vi "Final Shutdown.vi"(8 "error in (no error)":errorcluster, 11 "Main Controller in":refnum<class "Main Controller Actor.lvclass">) -> (0 "error out":errorcluster)   [LabVIEW 2021, in "Main Controller Actor.lvclass"]
uses:
  Main Controller Actor.lvclass
  Main Controller Actor.lvclass/Main Controller Actor.ctl
  Error Handler/API/Error Handler Actor API.lvclass
  Sprite Font/Sprite Font.lvclass
  Re-use Libraries/Minimal Actor Framework/Actors/Base Actor/API/Actor API.lvclass
  Task Scheduler/API/Task Scheduler Actor API.lvclass
  Element/Element.lvclass
  Globals.vi
  Re-use Libraries/Minimal Actor Framework/Actors/Base Actor/Actor/Actor.lvclass
  LabBASSMOD2/LabBASSMOD2.lvlib
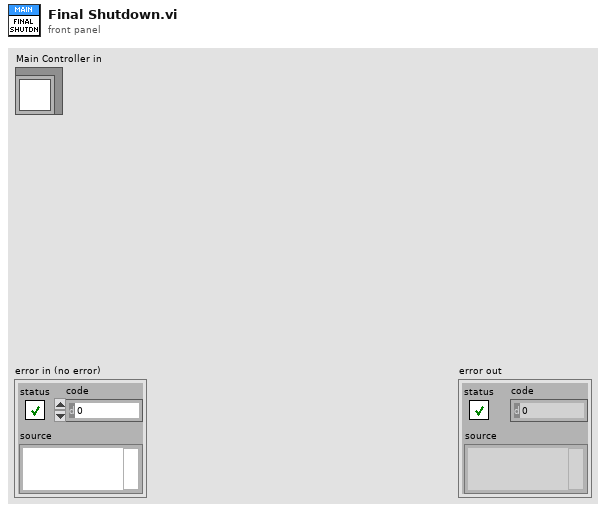
[diagram p1: front panel]
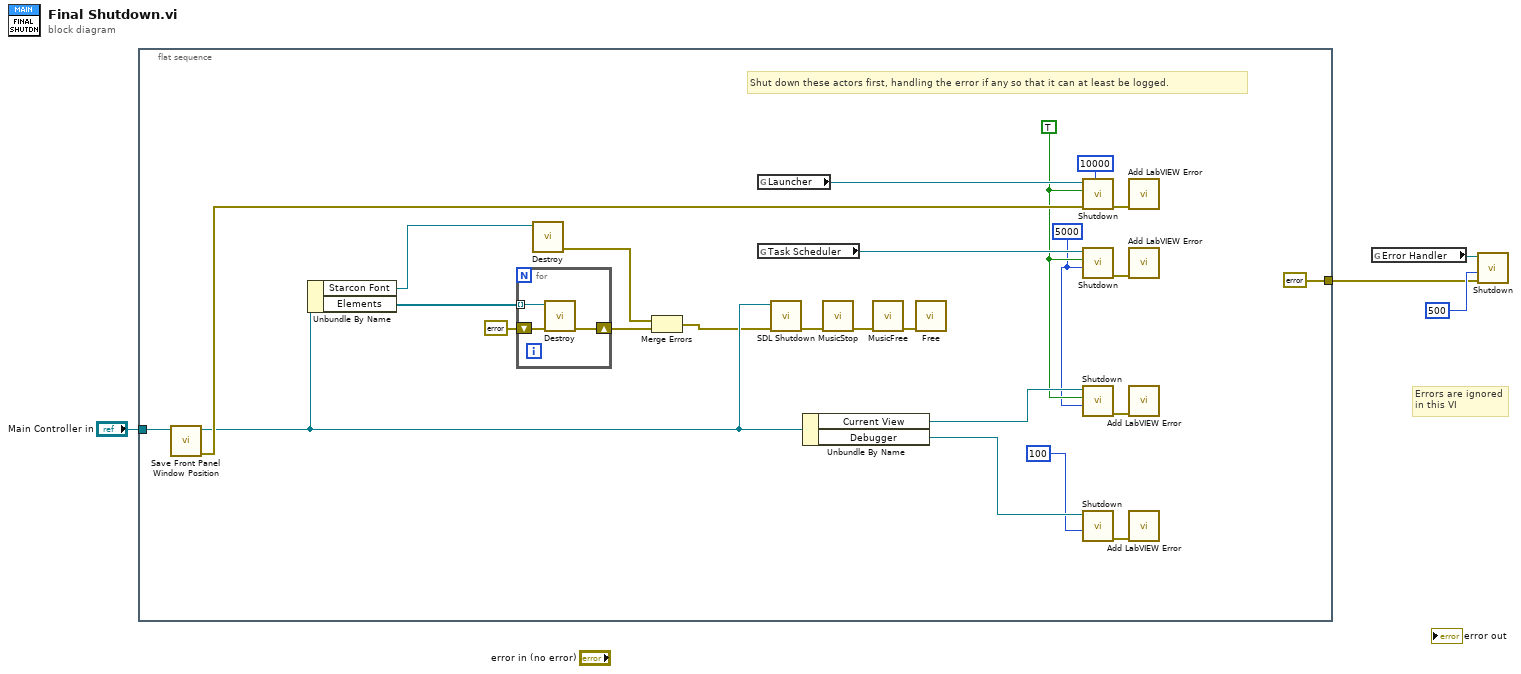
[diagram p0: block diagram]
diagram:
  # "Errors are ignored in this VI"
  n1 = flat-sequence {
    tunnel: "Main Controller in" -> [w9]
    tunnel: [errorcluster {"status"=FALSE, "code"=0, "source"=""} ("error constant")] -> w1
    frame #0 {
      w15 = 5000 ("Wait Timeout [10000 ms]")
      w16 = TRUE
      # "Shut down these actors first, handling the error if any so that it can at least be logged."
      n2 = call "Save Front Panel Window Position.vi"("Actor in"=w9) -> ("error out"=w24:errorcluster)  [unwired: 10 in]
      n3 = Unbundle By Name(w9) -> ("Starcon Font"=w8:refnum<class "Sprite Font.lvclass">, "Elements"=w11:refnum<class "Element.lvclass">[])
      n4 = for {
        tunnel: w11 -> [w29] mode=indexing
        shift-right: [w31] -> w7
        shift-left: errorcluster {"status"=FALSE, "code"=0, "source"=""} ("error out") -> [w30]
        n5 = call-dynamic "Destroy.vi"("error in (no error)"=w30, "Element in"=w29) -> ("error out"=w31:errorcluster)  [unwired: 9 in]
      }
      n6 = call-dynamic "Destroy.vi"("Font in"=w8) -> ("error out"=w5:errorcluster)  [unwired: 10 in]
      n7 = Merge Errors(w5, w7) -> (w6:errorcluster)
      n8 = global read "Globals.vi" "Launcher"() -> (w27:refnum<class "Actor API.lvclass">)
      n9 = global read "Globals.vi" "Task Scheduler"() -> (w25:refnum<class "Task Scheduler Actor API.lvclass">)
      n10 = call "SDL Shutdown.vi"("error in (no error)"=w6, "Main Controller Actor in"=w9) -> ("error out"=w10:errorcluster)  [unwired: 8 in, 1 out]
      n11 = Unbundle By Name(w9) -> ("Current View"=w28:refnum<class "Actor API.lvclass">, "Debugger"=w18:refnum<class "Actor API.lvclass">)
      n12 = call "MusicStop.vi"("error in (no error)"=w10) -> ("error out"=w12:errorcluster)  [unwired: 10 in]
      n13 = call "MusicFree.vi"("error in (no error)"=w12) -> ("error out"=w13:errorcluster)  [unwired: 10 in]
      n14 = call "Free.vi"("error in (no error)"=w13) -> ()  [unwired: 10 in, 1 out]
      n15 = call-dynamic "Shutdown.vi"("error in (no error)"=w24, "Wait Timeout [10000 ms]"=10000, "Wait For Shutdown (F)"=w16, "Actor API in"=w27) -> ("error out"=w22:errorcluster)  [unwired: 7 in]
      n16 = call-dynamic "Shutdown.vi"("Wait Timeout [10000 ms]"=w15, "Wait For Shutdown (F)"=w16, "Actor API in"=w25) -> ("error out"=w21:errorcluster)  [unwired: 8 in]
      n17 = call-dynamic "Shutdown.vi"("Wait Timeout [10000 ms]"=w15, "Wait For Shutdown (F)"=w16, "Actor API in"=w28) -> ("error out"=w20:errorcluster)  [unwired: 8 in]
      n18 = call-dynamic "Shutdown.vi"("Wait Timeout [10000 ms]"=100, "Actor API in"=w18) -> ("error out"=w19:errorcluster)  [unwired: 9 in]
      n19 = call "Add LabVIEW Error.vi"("error in (no error)"=w22) -> ()  [unwired: 10 in, 1 out]
      n20 = call "Add LabVIEW Error.vi"("error in (no error)"=w21) -> ()  [unwired: 10 in, 1 out]
      n21 = call "Add LabVIEW Error.vi"("error in (no error)"=w20) -> ()  [unwired: 10 in, 1 out]
      n22 = call "Add LabVIEW Error.vi"("error in (no error)"=w19) -> ()  [unwired: 10 in, 1 out]
    }
  }
  n23 = global read "Globals.vi" "Error Handler"() -> (w4:refnum<class "Error Handler Actor API.lvclass">)
  n24 = call-dynamic "Shutdown.vi"("error in (no error)"=w1, "Wait Timeout [10000 ms]"=500, "Actor API in"=w4) -> ()  [unwired: 8 in, 1 out]
